vi "get item properties.vi"(8 "error in (no error)":errorcluster, 11 "Device Ref in":T1 format="%.0x") -> (0 "error out":errorcluster, 1 "RIO target":string, 2 "heat params and ambient temp":dbl[](array[numeric]), 3 "thermal model rate":dbl, 4 "Path":path)   [LabVIEW 2014, in "UEGO Sim Engine.lvlib"]
uses:
  UEGO Sim Engine.lvlib
  <vilib>/NI Veristand/Custom Device API/Custom Device Item Ref.ctl
  Shared/Constants.vi
  <vilib>/NI Veristand/Custom Device API/Get Item Property (Double).vi
  <vilib>/NI Veristand/Custom Device API/Get Item Property (String).vi
  <vilib>/NI Veristand/Custom Device API/Get Item Property (Dependent File).vi
  <vilib>/NI Veristand/Custom Device API/Custom Device API.lvlib
  Shared/UEGO Sim Shared.lvlib
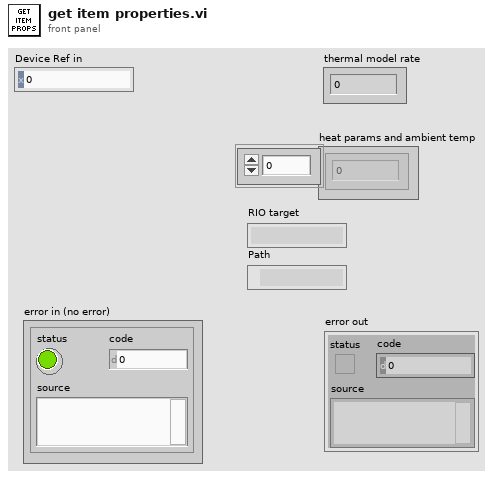
[diagram p1: front panel]
types:
  T1 = typedef "Custom Device API.lvlib/Custom Device Item Ref.ctl" = u64
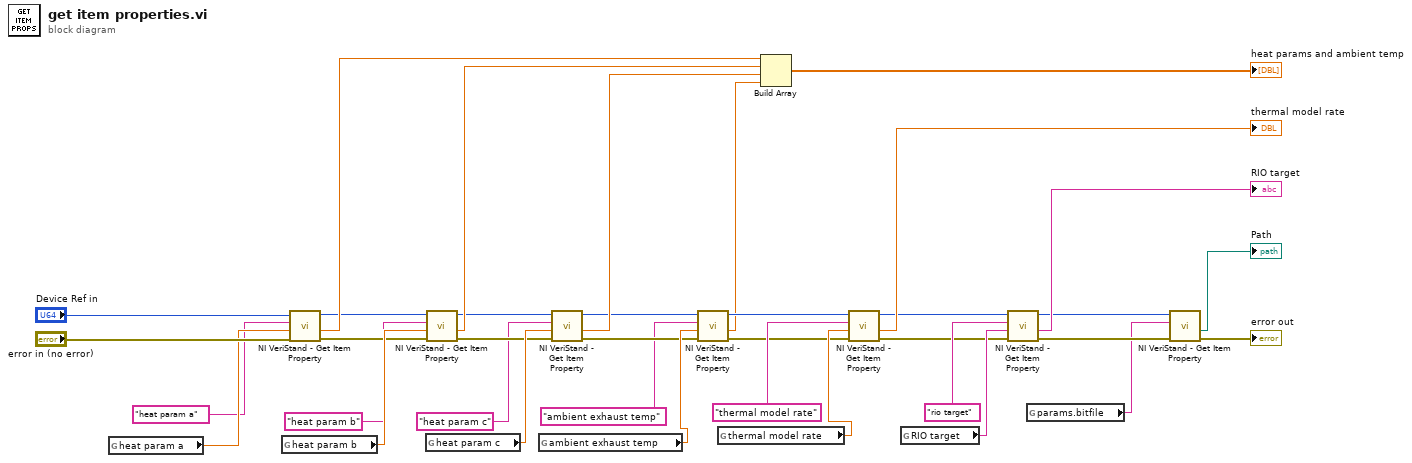
[diagram p0: block diagram]
diagram:
  n1 = global read "Constants.vi" "heat param a"() -> (w21:dbl)
  n2 = global read "Constants.vi" "heat param b"() -> (w22:dbl)
  n3 = call-poly <vilib>:"NI VeriStand - Get Item Property.vi"("error in (no error)"="error in (no error)", "Default Value"=w21, "Property Name"="heat param a", "Item Ref in"="Device Ref in") -> ("error out"=w14:errorcluster, "Value"=w29:dbl, "Item Ref out"=w13:T1)  [unwired: 4 in, 1 out]
  n4 = global read "Constants.vi" "heat param c"() -> (w23:dbl)
  n5 = call-poly <vilib>:"NI VeriStand - Get Item Property.vi"("error in (no error)"=w14, "Default Value"=w22, "Property Name"="heat param b", "Item Ref in"=w13) -> ("error out"=w17:errorcluster, "Value"=w28:dbl, "Item Ref out"=w16:T1)  [unwired: 4 in, 1 out]
  n6 = global read "Constants.vi" "ambient exhaust temp"() -> (w24:dbl)
  n7 = call-poly <vilib>:"NI VeriStand - Get Item Property.vi"("error in (no error)"=w17, "Default Value"=w23, "Property Name"="heat param c", "Item Ref in"=w16) -> ("error out"=w20:errorcluster, "Value"=w27:dbl, "Item Ref out"=w19:T1)  [unwired: 4 in, 1 out]
  n8 = call-poly <vilib>:"NI VeriStand - Get Item Property.vi"("error in (no error)"=w20, "Default Value"=w24, "Property Name"="ambient exhaust temp", "Item Ref in"=w19) -> ("error out"=w32:errorcluster, "Value"=w30:dbl, "Item Ref out"=w33:T1)  [unwired: 4 in, 1 out]
  n9 = global read "Constants.vi" "thermal model rate"() -> (w34:dbl)
  n10 = Build Array(w29, w28, w27, w30) -> (→"heat params and ambient temp":dbl[])
  n11 = call-poly <vilib>:"NI VeriStand - Get Item Property.vi"("error in (no error)"=w32, "Default Value"=w34, "Property Name"="thermal model rate", "Item Ref in"=w33) -> ("error out"=w7:errorcluster, "Value"=→"thermal model rate":dbl, "Item Ref out"=w8:T1)  [unwired: 4 in, 1 out]
  n12 = global read "Constants.vi" "RIO target"() -> (w10:string)
  n13 = call-poly <vilib>:"NI VeriStand - Get Item Property.vi"("error in (no error)"=w7, "Default Value"=w10, "Property Name"="rio target", "Item Ref in"=w8) -> ("error out"=w4:errorcluster, "Value"=→"RIO target":string, "Item Ref out"=w5:T1)  [unwired: 4 in, 1 out]
  n14 = global read "Constants.vi" "params.bitfile"() -> (w3:string)
  n15 = call-poly <vilib>:"NI VeriStand - Get Item Property.vi"("error in (no error)"=w4, "Property Name"=w3, "Item Ref in"=w5) -> ("error out"=→"error out":errorcluster, "Path"=→"Path":path)  [unwired: 4 in, 3 out]
